vi "trio_setvr_float.vi"(6 "Error/Warning (Error)":bool, 8 "error in (no error)":errorcluster, 9 "Value":dbl, 10 "Vr #":i16, 11 "reference in":refnum<k7>) -> (0 "error out":errorcluster, 3 "reference out":refnum<k7>, 5 "Vr Set":bool)   [LabVIEW 2017]
uses:
  <instrlib>/Trio Motion/Trio Motion Library.lvlib
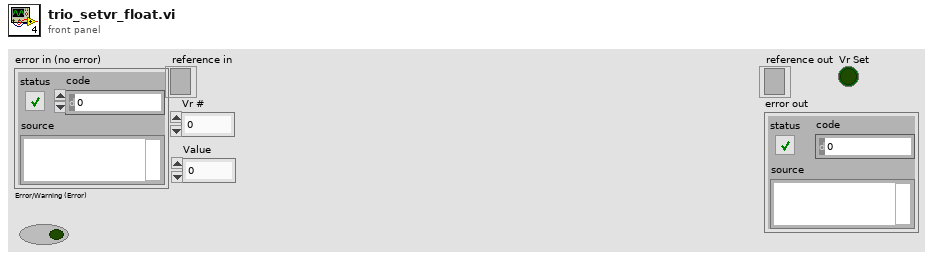
[diagram p1: front panel]
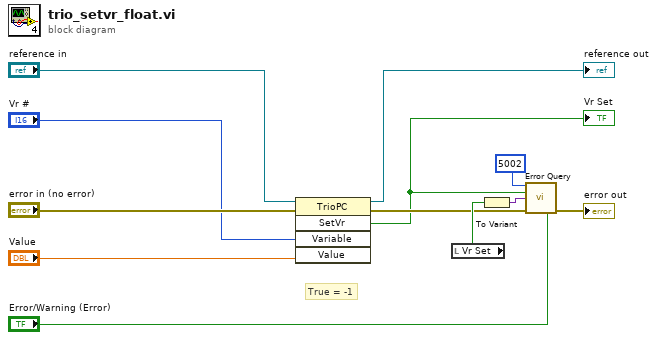
[diagram p0: block diagram]
diagram:
  # "True = -1"
  n1 = invoke class="TrioPC" method="SetVr"(reference="reference in", error in="error in (no error)", "Variable"="Vr #", "Value"="Value") -> (reference out=→"reference out":refnum<k7>, error out=w5:errorcluster, "SetVr"=w3:bool)  [unwired: 1 in, 2 out]
  "Vr Set" <- w3
  n2 = local read "Vr Set"() -> (w7:bool)
  n3 = To Variant(anything=w7) -> (Variant=w6:variant)
  n4 = call <instrlib>:"Error Query.vi"("error code (0)"=5002, "State"=w3, "Command"=w6, "error in (no error)"=w5, "Error/Warning (Error)"="Error/Warning (Error)") -> ("error out"=→"error out":errorcluster)  [unwired: 10 in]
